vi "mod_Generate doppler filter input.vi"(0 "profile length (samples)":i32=1000, 5 "standard deviation":dbl=1.0, 9 "seed in (0xFFFFFFFF)":i32=-1 format="%.0x", 11 "error in (no error)":errorcluster, 13 "reset? (T)":bool=TRUE) -> (4 "doppler filter input":cdb[](array[numeric]), 10 "seed out":i32 format="%.0x", 15 "error out":errorcluster)   [LabVIEW 2020, in "niDMT.lvlib"]
uses:
  <vilib>/addons/Modulation/niDMT.lvlib
  <vilib>/addons/Modulation/Digital/General/subVIs/mod_Generate Bits PN Sequence.vi
  <vilib>/Analysis/NI_AALBase.lvlib
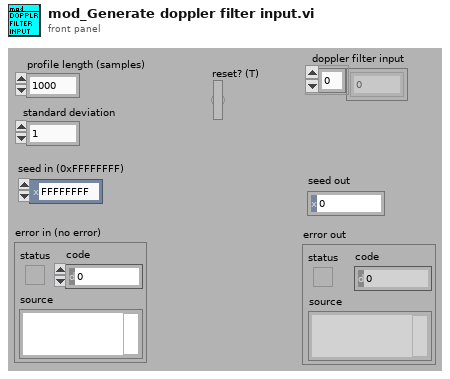
[diagram p1: front panel]
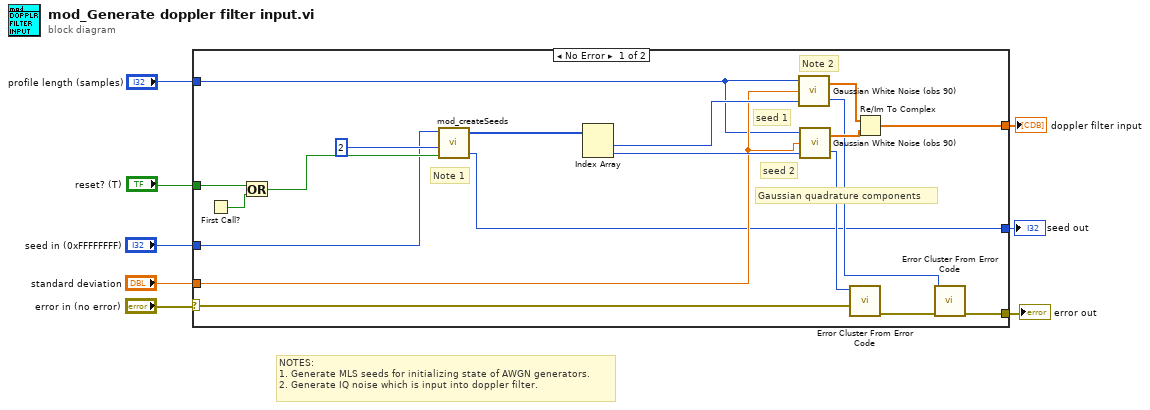
[diagram p0: block diagram]
diagram:
  # "NOTES:\n1. Generate MLS seeds for initializing state of AWGN generators.\n2. Generate IQ noise which is input into doppler filter."
  n1 = case shown="No Error" "error in (no error)" {
    selector: "error in (no error)" -> [w18 w28]
    tunnel: [w16 w28] -> w7
    tunnel: "profile length (samples)" -> [w10 _]
    tunnel: "reset? (T)" -> [w14 _]
    tunnel: "seed in (0xFFFFFFFF)" -> [w13 _]
    tunnel: "standard deviation" -> [w12 _]
    tunnel: [w11 _] -> w2
    tunnel: [w9 _] -> w1
    frame No Error {
      # "Note 2"
      # "Note 1"
      # "seed 2"
      # "seed 1"
      # "Gaussian quadrature components"
      n2 = First Call?() -> (First Call?: T/F=w23:bool)
      n3 = Or(x=w14, y=w23) -> (x .or. y?=w15:bool)
      n4 = call <vilib>:"mod_createSeeds.vi"("Reset? (T)"=w15, "# of seeds to create"=u32 2, "seed in (0xFFFFFFFF)"=w13) -> ("Next seed"=w9:i32, "Seeds"=w27:i32[])  [unwired: 1 in, 1 out]
      n5 = Index Array(array=w27) -> (element #1=w26:i32, element #2=w24:i32)  [unwired: 2 in]
      n6 = call <vilib>:"Gaussian White Noise (obs 90).vi"("seed"=w26, "standard deviation"=w12, "samples"=w10) -> ("error"=w20:i32, "Gaussian noise pattern"=w22:dbl[])
      n7 = call <vilib>:"Gaussian White Noise (obs 90).vi"("seed"=w24, "standard deviation"=w12, "samples"=w10) -> ("error"=w19:i32, "Gaussian noise pattern"=w21:dbl[])
      n8 = call <vilib>:"Error Cluster From Error Code.vi"("error in (no error)"=w18, "error code (0)"=w19) -> ("error out"=w17:errorcluster)  [unwired: 1 in, 6 out]
      n9 = Re/Im To Complex(1:w21, 2:w22) -> (0:w11:cdb[])
      n10 = call <vilib>:"Error Cluster From Error Code.vi"("error in (no error)"=w17, "error code (0)"=w20) -> ("error out"=w16:errorcluster)  [unwired: 1 in, 6 out]
    }
    frame Error {
    }
  }
  "error out" <- w7
  "doppler filter input" <- w2
  "seed out" <- w1
